vi "串口直接读写C71-FA波特率57600_简化数值.vi"(0 "VISA resource name":refnum<visa-resource-name>="COM8" caption="VISA资源名称") -> ()   [LabVIEW 2020]
doc: "基本串口读取和写入范例可实现串口读取、串口写入或者串口读写操作。用户可在前面板选择操作（读取或写入）。如果选择全部，VI将写入数据并读取数据，然后关闭开放给端口的VISA会话句柄。该VI将等待直到端口接收到指定的字节数。\n\n操作步骤：\n1) 选择串行资源并配置参数（波特率、数据位、奇偶、停止位和流控制）。\n2) 选择需执行的操作。\n3) 连接串口至设备。如未发现可用设备，请按以下任一方式执行环回测试。在RS-232线缆中短路引脚2和3，或者在RS-485/422线缆中短路引脚4和8以及引脚5和9。\n4) 运行VI并查看读取的数据。（如果已执行环回测试，“读取字符串”将匹配“写入字符串”。）\n\n注：串口的参数组必须匹配连接仪器或设备的参数。在本范例中，待读取字节参数可指定串口读取的字节数。如端口字节超过指定的字节数，超出部分将不会被读取。如果指定读取的字节数超过实际字节数，可能返回超时错误。\n\n在程序框图中，“配置串口VI”可用于设置配置参数。前面板显示的控件可用于配置基本参数，如波特率、数据位和奇偶。常量可配置其它用户无需设置的参数。“VISA配置串口VI”打开VISA句柄并配置端口后，该VI会将VISA资源名称传递至其它VI以便执行相关操作。“VISA写入”函数将发送一个命令至串行设备，“VISA读取”函数将返回基于该命令的数据。“VISA关闭”函数可关闭该串行设备的引用。关闭引用十分重要，否则可能导致VISA无法通过端口和协议进行通信。"
uses:
  <vilib>/Instr/_visa.llb/VISA Configure Serial Port (Instr).vi
panel:
  out "读取缓冲区":string
  out "延时（ms）":u32
  out "值":dbl
  in  "停止":bool
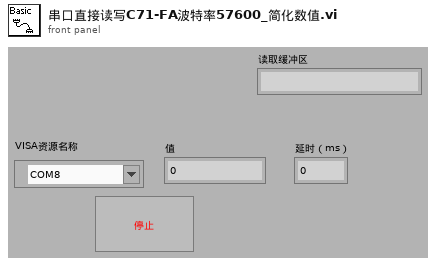
[diagram p1: front panel]
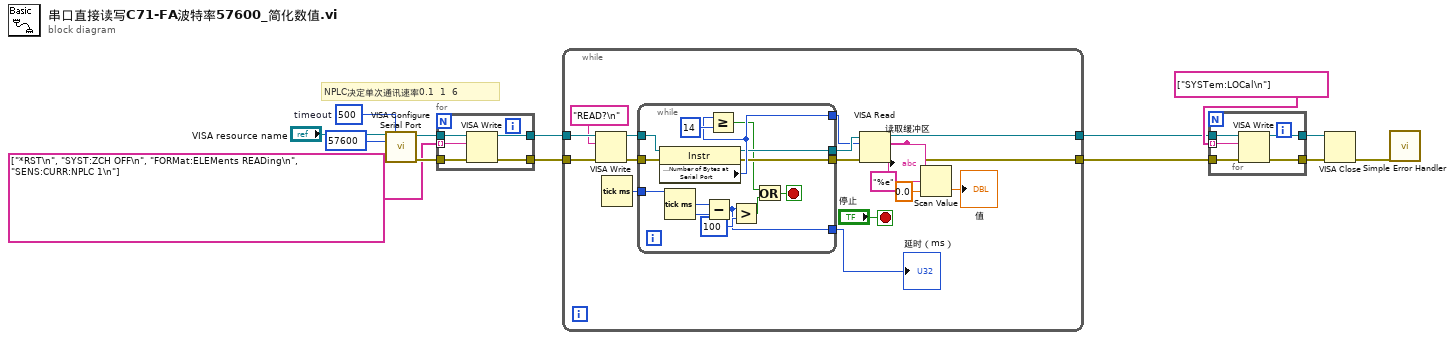
[diagram p0: block diagram]
diagram:
  w11 = u32 500  # timeout
  # "NPLC决定单次通讯速率0.1  1  6"
  n1 = call-poly "VISA Configure Serial Port"("VISA resource name"="VISA resource name", "timeout (10sec)"=w11, "baud rate (9600)"=u32 57600 ("baud rate")) -> ("VISA resource name out"=w10:refnum<visa-resource-name>, "error out"=w9:errorcluster)  [unwired: 6 in, 5 out]
  n2 = for {
    tunnel: w10 -> [w19]
    tunnel: w9 -> [w18]
    tunnel: [w17] -> w8
    tunnel: [w16] -> w7
    tunnel: string[] ["*RST\n", "SYST:ZCH OFF\n", "FORMat:ELEMents READing\n", "SENS:CURR:NPLC 1\n"] -> [w15] mode=indexing
    n3 = VISA Write(VISA resource name=w19, write buffer=w15, error in (no error)=w18) -> (VISA resource name out=w17:refnum<visa-resource-name>, error out=w16:errorcluster)  [unwired: 1 out]
  }
  n4 = while {
    tunnel: w7 -> [w36]
    tunnel: w8 -> [w35]
    tunnel: [w34] -> w4
    tunnel: [w33] -> w5
    stop <- "停止" stop-if-true
    n5 = VISA Write(VISA resource name=w35, write buffer="READ?\n" ("string to write"), error in (no error)=w36) -> (VISA resource name out=w30:refnum<visa-resource-name>, error out=w32:errorcluster)  [unwired: 1 out]
    n6 = Tick Count (ms)() -> (millisecond timer value=w25:u32)
    n7 = while {
      tunnel: [w48] -> w27
      tunnel: w30 -> [w47]
      tunnel: w32 -> [w46]
      tunnel: [w45] -> w29
      tunnel: [w44] -> w31
      tunnel: w25 -> [w42]
      tunnel: [w37] -> w20
      stop <- w39 stop-if-true
      n8 = property class="Instr"(reference=w47, error in=w46) -> (reference out=w45:refnum<visa-resource-name>, error out=w44:errorcluster, "Serial Settings:Number of Bytes at Serial Port"=w48:u32)
      n9 = Tick Count (ms)() -> (millisecond timer value=w43:u32)
      n10 = Subtract(x=w43, y=w42) -> (x-y=w37:u32)
      n11 = Greater Or Equal?(x=w48, y=u32 14) -> (x >= y?=w40:bool)
      n12 = Greater?(x=w37, y=u32 100) -> (0:w38:bool)
      n13 = Or(x=w40, y=w38) -> (x .or. y?=w39:bool)
    }
    "延时（ms）" <- w20
    n14 = VISA Read(VISA resource name=w29, byte count=w27, error in (no error)=w31) -> (VISA resource name out=w33:refnum<visa-resource-name>, read buffer=w22:string, error out=w34:errorcluster)  [unwired: 1 out]
    "读取缓冲区" <- w22
    n15 = Scan Value(string=w22, format string="%e" ("格式字符串"), default (0 dbl)=0.0 ("默认(0 dbl)")) -> (value=→"值":dbl)  [unwired: 1 out]
  }
  n16 = for {
    tunnel: w5 -> [w54]
    tunnel: w4 -> [w53]
    tunnel: [w52] -> w3
    tunnel: [w51] -> w2
    tunnel: string[] ["SYSTem:LOCal\n"] -> [w50] mode=indexing
    n17 = VISA Write(VISA resource name=w54, write buffer=w50, error in (no error)=w53) -> (VISA resource name out=w52:refnum<visa-resource-name>, error out=w51:errorcluster)  [unwired: 1 out]
  }
  n18 = VISA Close(VISA resource name=w3, error in (no error)=w2) -> (error out=w12:errorcluster)
  n19 = call <vilib>:"Simple Error Handler.vi"("error in (no error)"=w12) -> ()  [unwired: 1 in, 8 out]
